vi "get_output_voltage.vi"(8 "error in (no error)":errorcluster, 11 "GenericAnalogOut in":refnum<class "GenericAnalogOut.lvclass">) -> (0 "error out":errorcluster, 2 "current voltage":dbl[unit], 3 "GenericAnalogOut out":refnum<class "GenericAnalogOut.lvclass">)   [LabVIEW 2010, in "GenericAnalogOut.lvclass"]
uses:
  GenericAnalogOut.lvclass
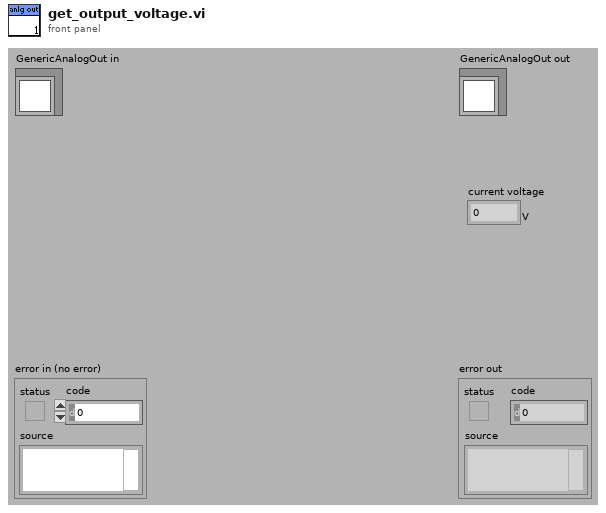
[diagram p1: front panel]
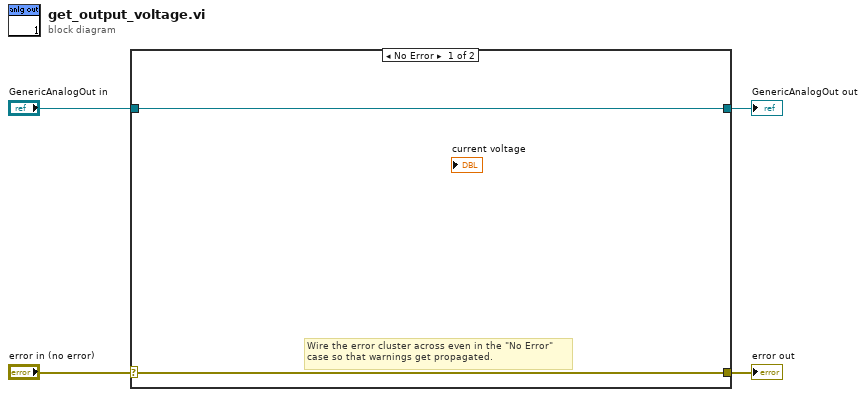
[diagram p0: block diagram]
diagram:
  n1 = case shown="No Error" "error in (no error)" {
    selector: "error in (no error)" -> [w5 w8]
    tunnel: [w5 w8] -> w3
    tunnel: [w6 w7] -> w1
    tunnel: "GenericAnalogOut in" -> [w6 w7]
    frame No Error {
      # "Wire the error cluster across even in the \"No Error\"\ncase so that warnings get propagated."
    }
    frame Error {
    }
  }
  "error out" <- w3
  "GenericAnalogOut out" <- w1
